vi "SaveCSV.vi"(6 "Data":string[][](array[string]), 7 "Save path":path=path "C:/Users/A. Halstesd Evander/Documents/VCU_BoxBuild/Info/DATA", 8 "error in (no error)":errorcluster, 9 "Tempelate path":path=path "C:/Users/A. Halstesd Evander/Documents/VCU_BoxBuild/Info/Configuration/Report_Template.csv", 10 "Summary Details":string[](array[string])=["1234", "Real_demo", "06-02-2025", "", "1", "Pass"], 11 "Filename":string="123.csv") -> (0 "error out":errorcluster, 2 "all rows":string[][](array[string]), 3 "CSVpath":path)   [LabVIEW 2024, in "Test_2.lvlib"]
uses:
  Test_2.lvlib
  <vilib>/Utility/file.llb/Read Delimited Spreadsheet (string).vi
  <vilib>/Utility/file.llb/Write Delimited Spreadsheet (string).vi
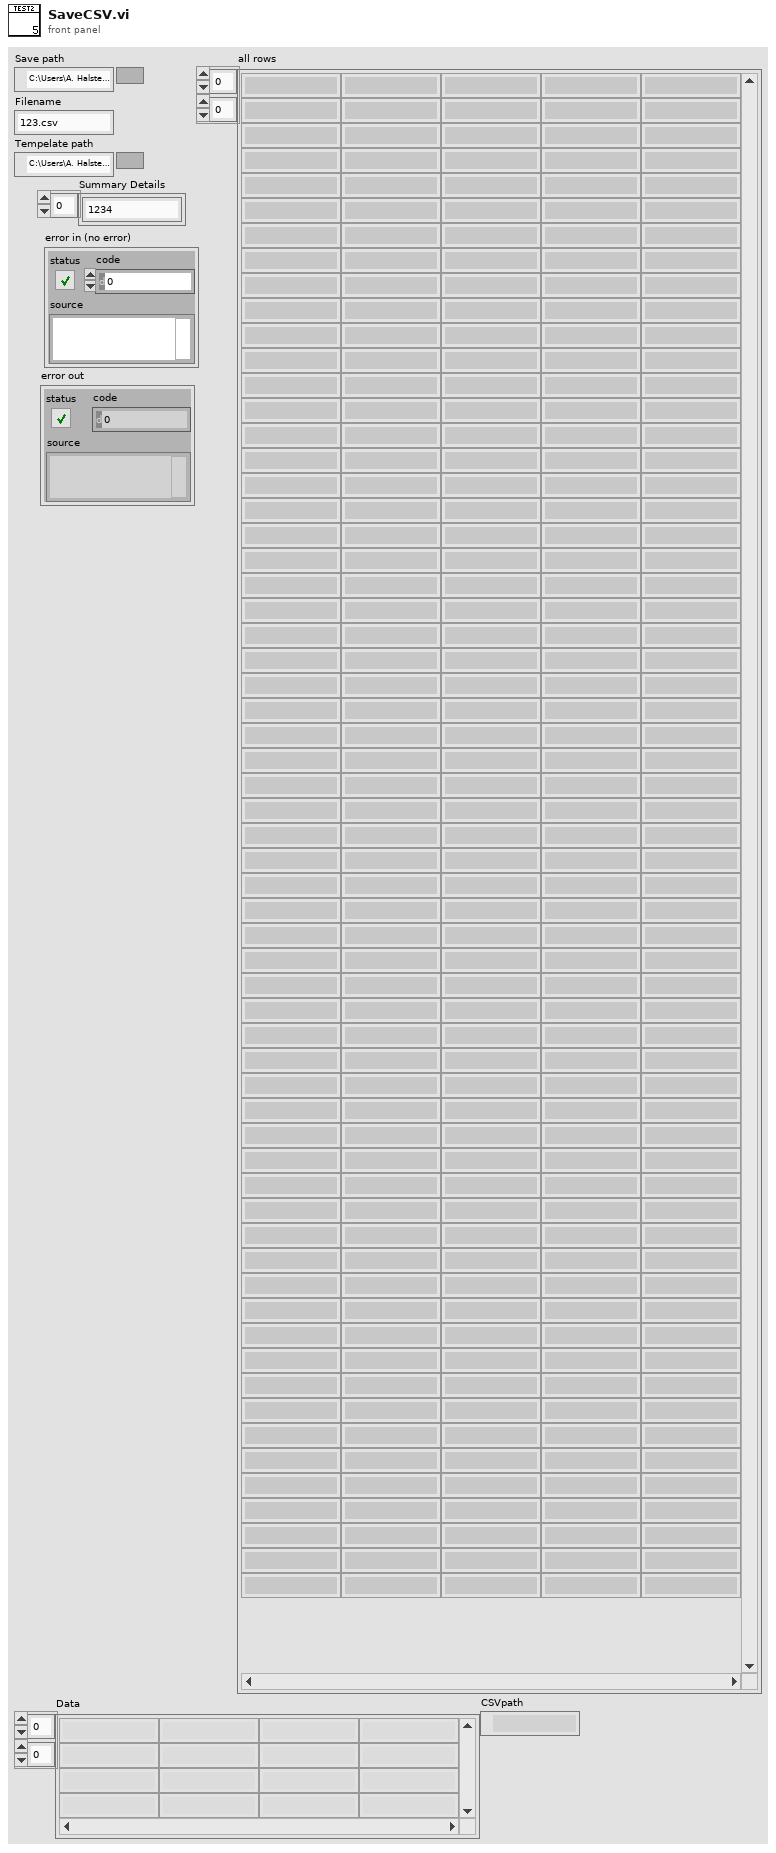
[diagram p1: front panel]
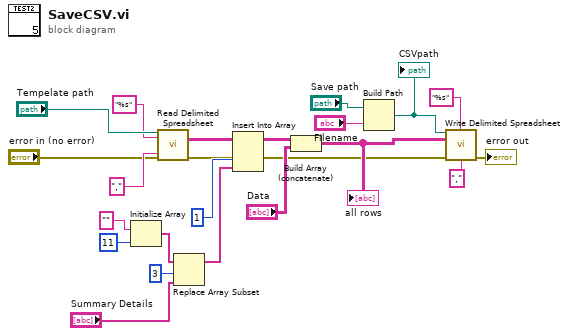
[diagram p0: block diagram]
diagram:
  n1 = Initialize Array("", 11 ("dimension size")) -> (w17:string[])
  n2 = call-poly <vilib>:"Read Delimited Spreadsheet.vi"("file path (dialog if empty)"="Tempelate path", "format (%s)"="%s", "error in (no error)"="error in (no error)", "delimiter (\\t)"="," ("delimiter (\\t)")) -> ("all rows"=w21:string[][], "error out"=w2:errorcluster)  [unwired: 6 in, 4 out]
  n3 = Replace Array Subset(array=w17, new element="Summary Details", index=3) -> (w14:string[])
  n4 = Insert Into Array(array=w21, index (col)=1 ("disabled index (col)"), new element=w14) -> (w11:string[][])  [unwired: 1 in]
  n5 = Build Array (concatenate)(w11, "Data") -> (w10:string[][])
  "all rows" <- w10
  n6 = Build Path(base path="Save path", name or relative path="Filename") -> (appended path=w5:path)
  "CSVpath" <- w5
  n7 = call-poly <vilib>:"Write Delimited Spreadsheet.vi"("file path (dialog if empty)"=w5, "format (%s)"="%s", "2D data"=w10, "error in (no error)"=w2, "delimiter (\\t)"="," ("delimiter (\\t)")) -> ("error out"=→"error out":errorcluster)  [unwired: 9 in, 1 out]
